vi "Decompose Variant.vi"(8 "error in (no error)":errorcluster, 11 "Arrray Variant":variant) -> (0 "error out":errorcluster, 3 "[Variant]":variant[](array[variant]))   [LabVIEW 2018, in "TwinCAT ADS.lvclass"]
uses:
  TwinCAT ADS.lvclass
  <vilib>/Utility/Data Type/NI_Data Type.lvlib
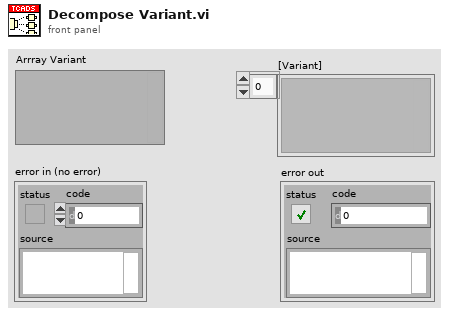
[diagram p1: front panel]
types:
  T1 = typedef "NI_Data Type.lvlib/Data Type.ctl" = enum8{"Invalid Type", "Void", "I8", "I16", "I32", "I64", "U8", "U16", "U32", "U64", "Single Float", "Double Float", "Extended Float", "Single Complex", "Double Complex", "Extended Complex", "Enum U8", "Enum U16", "Enum U32", "Enum U64", "Single Float With Unit", "Double Float With Unit", "Extended Float With Unit", "Single Complex with Unit", "Double Complex with Unit", "Extended Complex with Unit", "Boolean", "String", "Path", "Picture", "Tag", "Array", "Cluster", "Variant", "LV Variant", "Waveform", "Timestamp", "Digital Waveform", "Digital Data", "ExpressData", "Refnum", "External Data", "VI", "Poly VI", "LabVIEW Class Instance", "Fixed Point"}
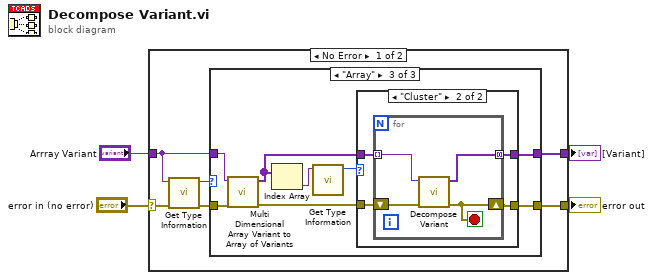
[diagram p0: block diagram]
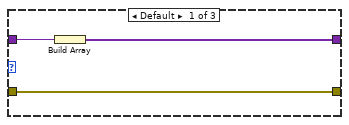
[diagram p2: hidden frame]
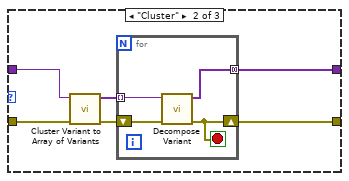
[diagram p3: hidden frame]
diagram:
  n1 = case shown="No Error" "error in (no error)" {
    selector: "error in (no error)" -> [w5 w42]
    tunnel: "Arrray Variant" -> [w9 _]
    tunnel: [w8 _] -> w3
    tunnel: [w6 w42] -> w2
    frame No Error {
      n2 = call <vilib>:"Get Type Information.vi"("error in (no error)"=w5, "Variant"=w9) -> ("error out"=w7:errorcluster, "Type"=w10:T1)  [unwired: 5 in, 3 out]
      n3 = case shown="\"Array\"" w10 {
        tunnel: w9 -> [w13 w16 w28]
        tunnel: [w12 w18 w31] -> w8
        tunnel: w7 -> [w11 w17 w29]
        tunnel: [w11 w19 w30] -> w6
        frame Default {
          n4 = Build Array(w13) -> (w12:variant[])
        }
        frame "Cluster" {
          n5 = call "Cluster Variant to Array of Variants.vi"("error in (no error)"=w17, "Cluster Variant"=w16) -> ("error out"=w15:errorcluster, "[Variant]"=w14:variant[])  [unwired: 8 in]
          n6 = for {
            tunnel: w14 -> [w23] mode=indexing
            shift-right: [w20] -> w19
            shift-left: w15 -> [w22]
            tunnel: [w21] -> w18 mode=concatenating
            stop <- w20 stop-if-true
            n7 = call "Decompose Variant.vi"("error in (no error)"=w22, "Arrray Variant"=w23) -> ("error out"=w20:errorcluster, "[Variant]"=w21:variant[])  [unwired: 8 in]
          }
        }
        frame "Array" {
          n8 = call "Multi Dimensional Array Variant to Array of Variants.vi"("error in (no error)"=w29, "Array Variant"=w28) -> ("error out"=w25:errorcluster, "[Variant]"=w26:variant[])  [unwired: 8 in]
          n9 = Index Array(array=w26) -> (element=w24:variant)  [unwired: 1 in]
          n10 = call <vilib>:"Get Type Information.vi"("Variant"=w24) -> ("Type"=w27:T1)  [unwired: 6 in, 4 out]
          n11 = case shown="\"Cluster\"" w27 {
            tunnel: w26 -> [w33 w37]
            tunnel: [w33 w35] -> w31
            tunnel: [w32 w34] -> w30
            tunnel: w25 -> [w32 w36]
            frame Default {
            }
            frame "Cluster" {
              n12 = for {
                tunnel: w37 -> [w41] mode=indexing
                shift-right: [w38] -> w34
                shift-left: w36 -> [w40]
                tunnel: [w39] -> w35 mode=concatenating
                stop <- w38 stop-if-true
                n13 = call "Decompose Variant.vi"("error in (no error)"=w40, "Arrray Variant"=w41) -> ("error out"=w38:errorcluster, "[Variant]"=w39:variant[])  [unwired: 8 in]
              }
            }
          }
        }
      }
    }
    frame Error {
    }
  }
  "[Variant]" <- w3
  "error out" <- w2
